vi "比较批次号关键字.vi"(8 "批次号":string, 9 "外购件名称":string, 10 "产品型号":string) -> (1 "关键字正确":bool, 3 "批次号 2":string)   [LabVIEW 2013]
panel:
  in  "error in (no error)":errorcluster
  out "error out":errorcluster
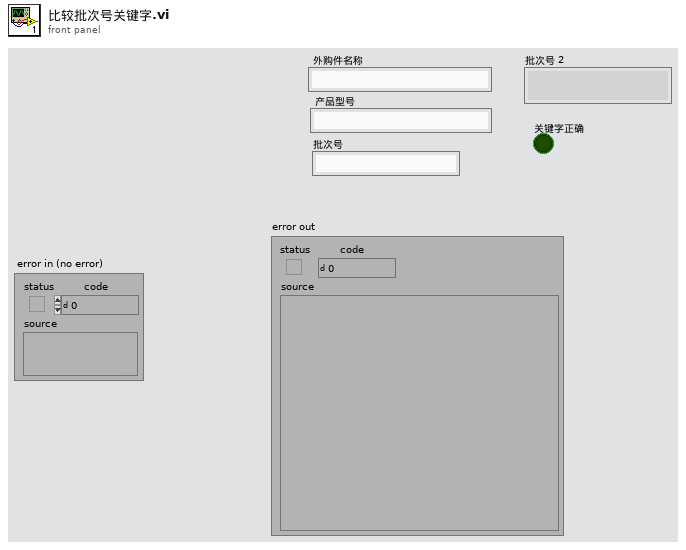
[diagram p1: front panel]
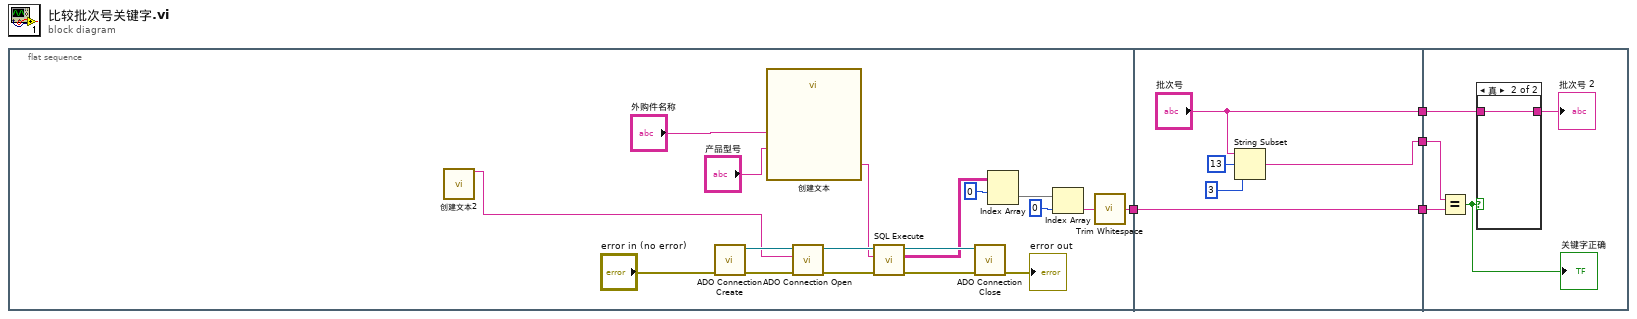
[diagram p0: block diagram]
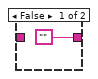
[diagram p2: hidden frame]
diagram:
  n1 = flat-sequence {
    tunnel: [w6] -> w3
    tunnel: [w23] -> w4
    tunnel: w3 -> [w27]
    tunnel: [w27] -> w2
    tunnel: ["批次号"] -> w1
    tunnel: w4 -> [w32]
    tunnel: w2 -> [w31]
    tunnel: w1 -> [w29]
    frame #0 {
      n2 = call "创建文本2"() -> ("Result"=w5:string)  [unwired: 14 in, 1 out]
      n3 = call "ADO Connection Create.vi"("error in (no error)"="error in (no error)") -> ("error out"=w21:errorcluster, "ADODB._Connection Out"=w22:refnum<k7>)  [unwired: 9 out]
      n4 = call "创建文本"("外购件名称"="外购件名称", "产品型号"="产品型号") -> ("Result"=w14:string)  [unwired: 12 in, 1 out]
      n5 = call "ADO Connection Open.vi"("error in (no error)"=w21, "ConnectionString"=w5, "ADODB._Connection In"=w22) -> ("error out"=w18:errorcluster, "ADODB._Connection Out"=w19:refnum<k7>)  [unwired: 7 out]
      n6 = call "SQL Execute.vi"("error in (no error)"=w18, "Command Text"=w14, "ADODB._Connection In"=w19) -> ("error out"=w16:errorcluster, "Data"=w11:string[][], "ADODB._Connection Out"=w17:refnum<k7>)  [unwired: 5 in, 1 out]
      n7 = call "ADO Connection Close.vi"("error in (no error)"=w16, "ADODB._Connection In"=w17) -> ("error out"=→"error out":errorcluster)  [unwired: 8 in, 1 out]
      n8 = Index Array(array=w11, index (row)=0 ("索引 (行)")) -> (element=w9:string[])  [unwired: 1 in]
      n9 = Index Array(array=w9, index=0 ("索引")) -> (element=w7:string)
      n10 = call <vilib>:"Trim Whitespace.vi"("string"=w7) -> ("trimmed string"=w6:string)  [unwired: 1 in]
    }
    frame #1 {
      n11 = String Subset(string="批次号", offset (0)=13 ("偏移量(0)"), length (rest)=3 ("长度（剩余）")) -> (substring=w23:string)
    }
    frame #2 {
      n12 = Equal?(x=w32, y=w31) -> (x = y?=w30:bool)
      "关键字正确" <- w30
      n13 = case shown="真" w30 {
        tunnel: w29 -> [_ w34]
        tunnel: ["" w34] -> w28
        frame False {
        }
        frame True {
        }
      }
      "批次号 2" <- w28
    }
  }
